vi "process-exe.vi"(0 "SR830 in":refnum<vi>, 1 "Monochromator":refnum<vi>, 3 "PowerGraph":refnum<vi>, 5 "Parameters":refnum<vi>, 9 "Process In":refnum<vi>, 11 "error in":errorcluster, 12 "Powermeter":refnum<vi>, 13 "Arr Power":refnum<vi>, 14 "Arr Refnum":refnum<vi>) -> (4 "Process out":refnum<vi>, 15 "error out":errorcluster)   [LabVIEW 2016]
uses:
  controls/process.ctl
  <vilib>/silver_ctls/ArrayMatrixCluster/Real Matrix NI_Silver.ctl
  <vilib>/Analysis/NI_AALBase.lvlib
panel:
  in  "PowerData":dbl[][](array[numeric])
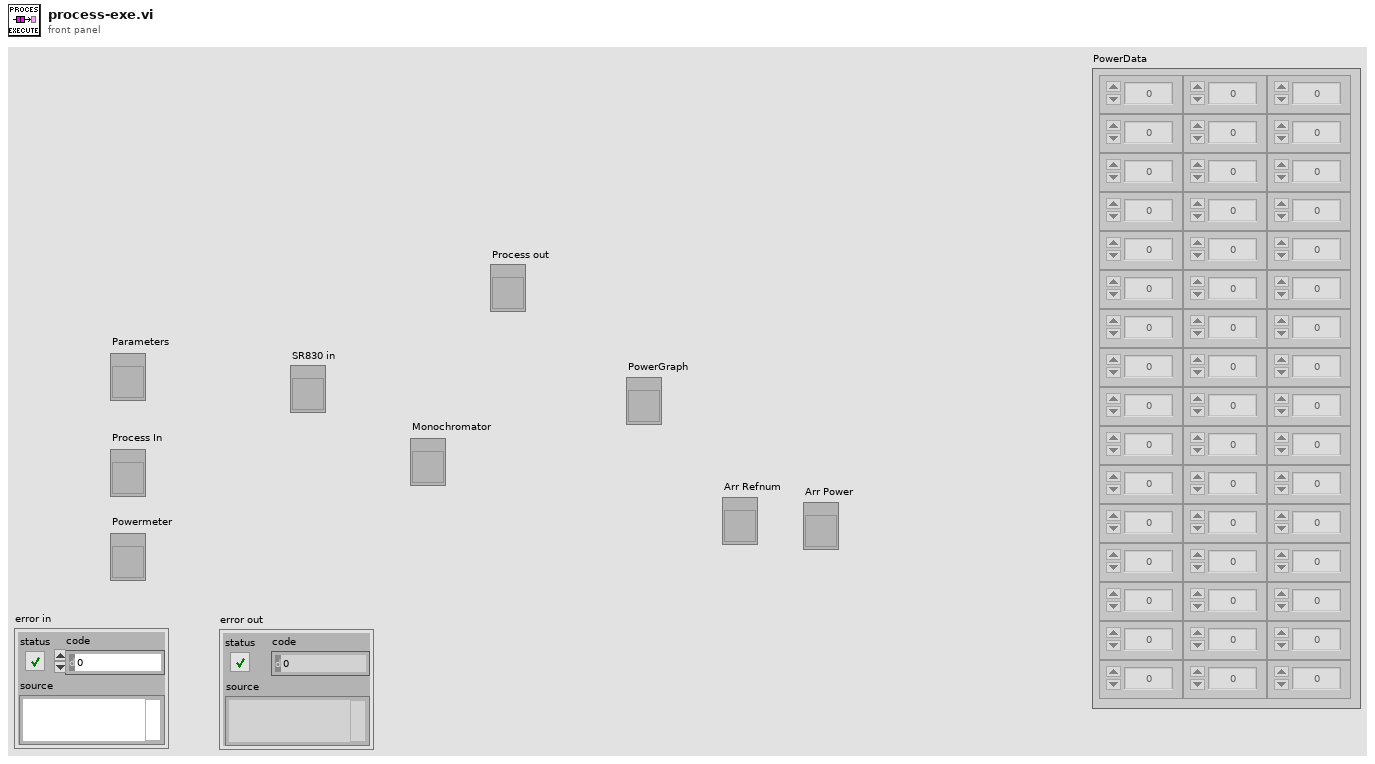
[diagram p1: front panel]
types:
  T1 = typedef "process.ctl" = cluster{"Sample":u16, "Lambda":u16, "Stabilizing":u16, "Status":u8, "Estimated Time":dbl, "Samples":T2, "Data":T2, "Lambda-Index":dbl, "Graph":bool}
  T2 = typedef "Real Matrix NI_Silver.ctl" = dbl[][]
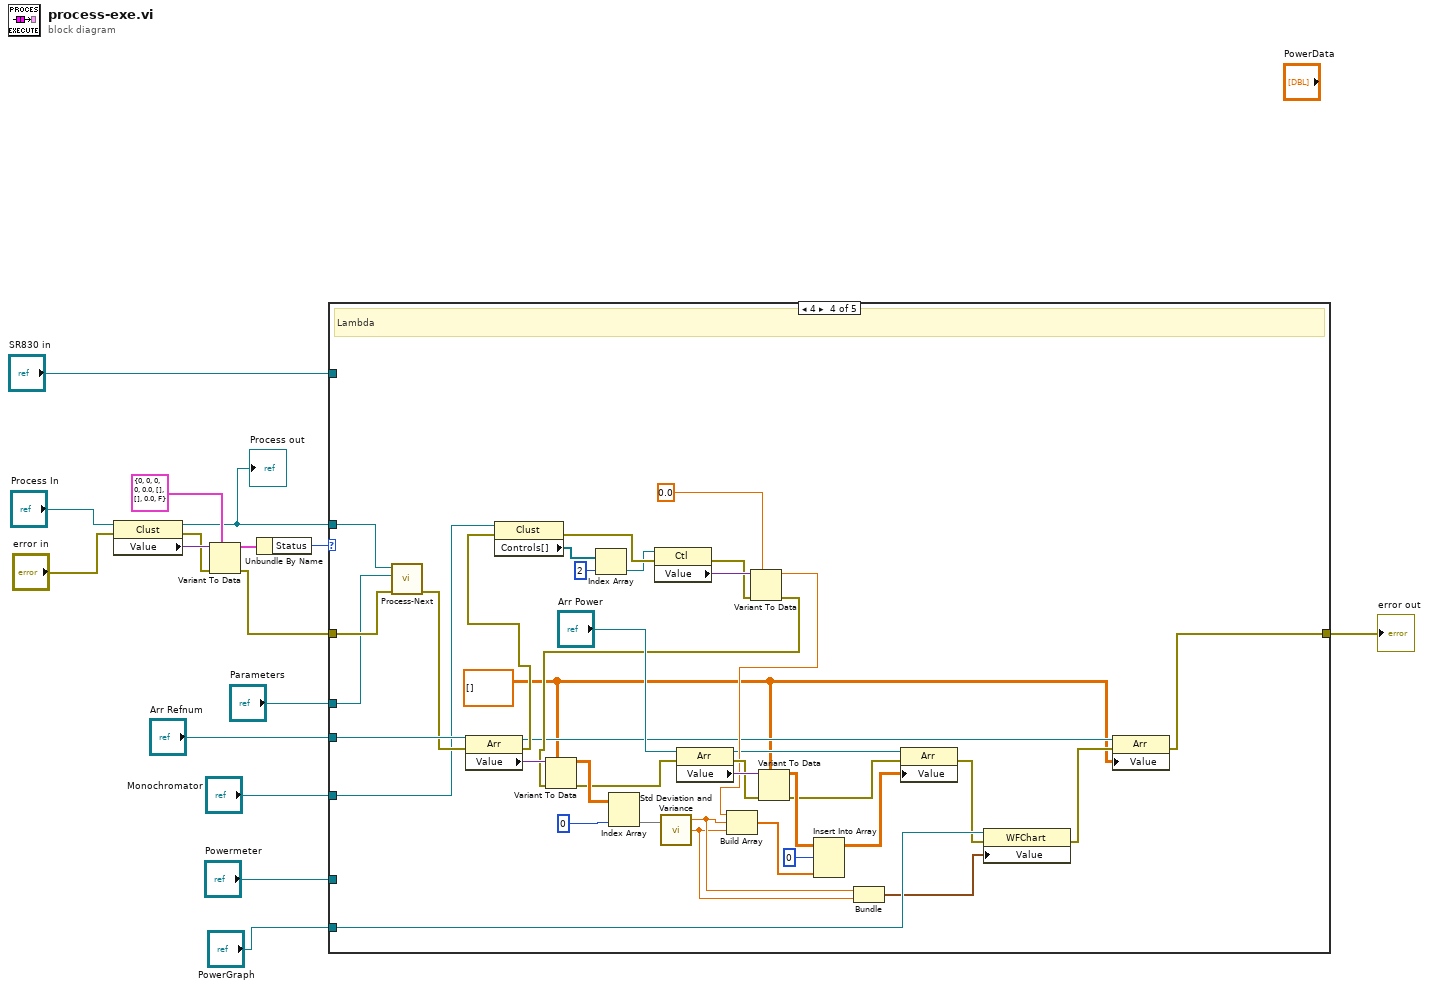
[diagram p0: block diagram]
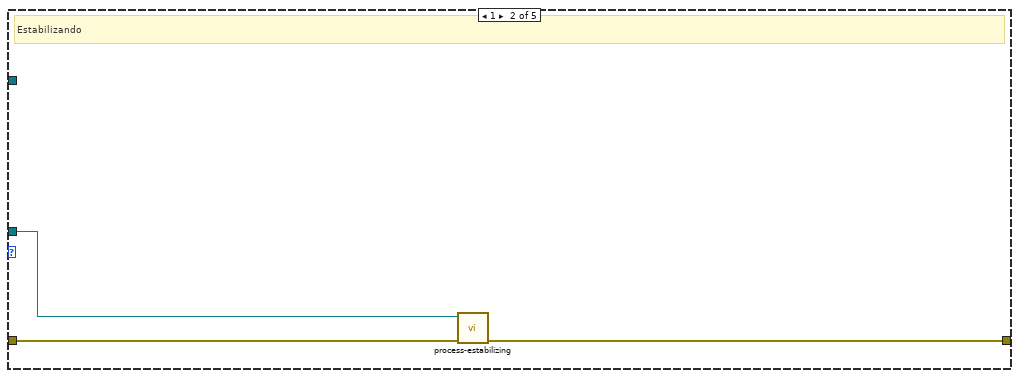
[diagram p3: hidden frame]
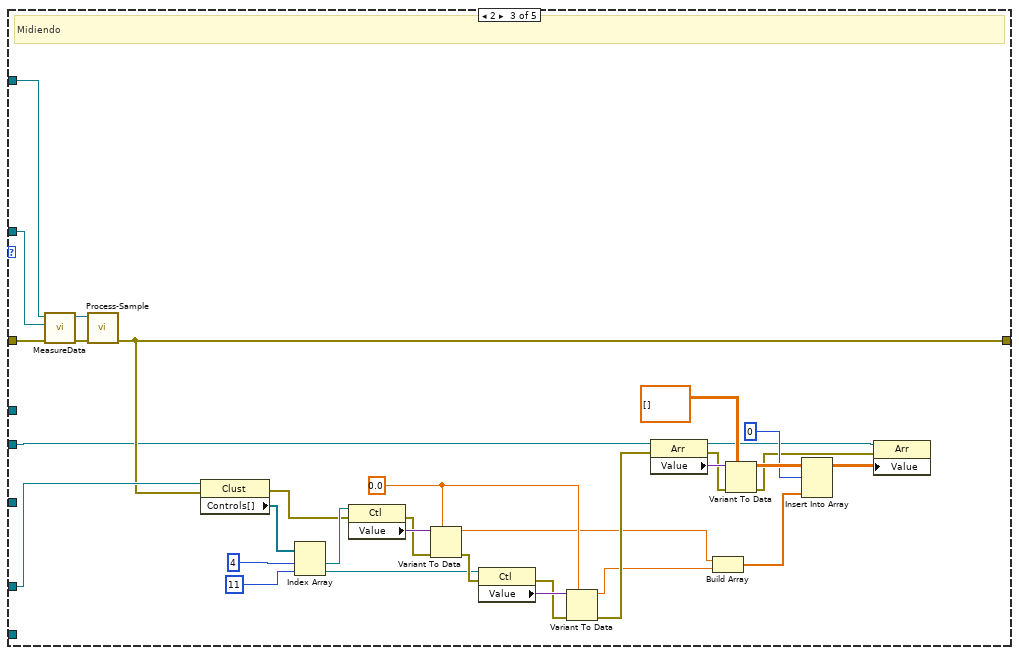
[diagram p4: hidden frame]
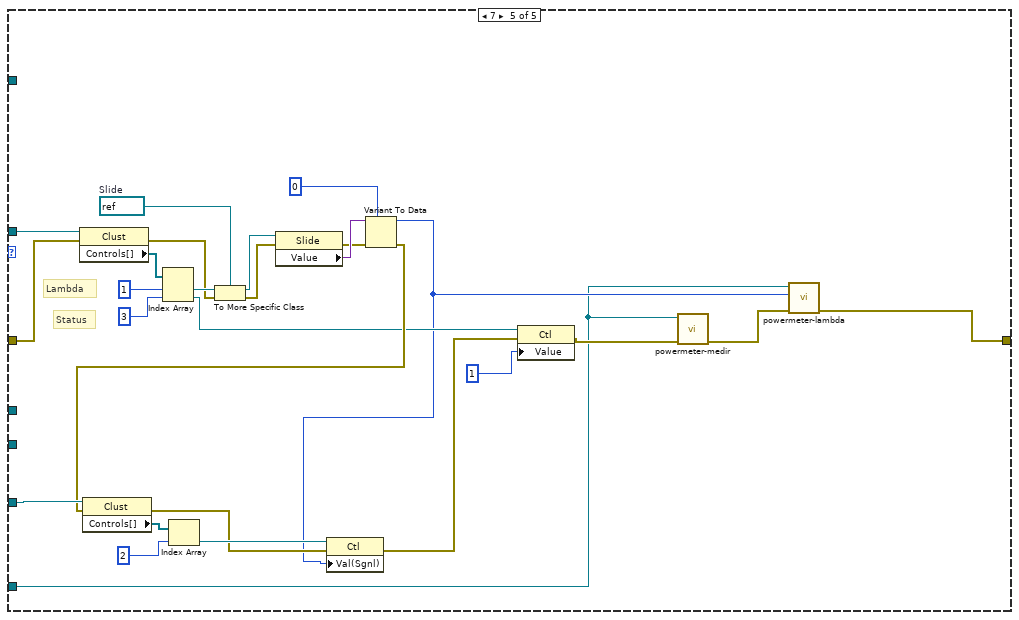
[diagram p5: hidden frame]
diagram:
  n1 = property class="Clust"(reference="Process In", error in="error in") -> (reference out=w7:refnum<vi>, error out=w13:errorcluster, "Value"=w14:variant)
  "Process out" <- w7
  n2 = Variant To Data(error in=w13, type=T1 {"Sample"=0, "Lambda"=0, "Stabilizing"=0, "Status"=0, "Estimated Time"=0.0, "Samples"=[], "Data"=[], "Lambda-Index"=0.0, "Graph"=FALSE} ("Process"), Variant=w14) -> (data=w11:T1, error out=w9:errorcluster)
  n3 = Unbundle By Name(w11) -> ("Status"=w10:u8)
  n4 = case shown="4" w10 {
    tunnel: w9 -> [w17 w20 w52 w91 w106]
    tunnel: [w17 w19 w46 w53 w96] -> w8
    tunnel: w7 -> [_ w18 w48 w65 w118]
    tunnel: "Parameters" -> [_ _ _ w90 _]
    tunnel: "SR830 in" -> [_ _ w49 _ _]
    tunnel: "Monochromator" -> [_ _ _ w66 w107]
    tunnel: "Powermeter" -> [_ _ w47 _ w92]
    tunnel: "Arr Refnum" -> [_ _ w33 w89 _]
    tunnel: "PowerGraph" -> [_ _ _ w61 _]
    frame 0, Default {
    }
    frame 1 {
      # "Estabilizando"
      n5 = call "process-estabilizing.vi"("error in (no error)"=w20, "Process in"=w18) -> ("error out"=w19:errorcluster)  [unwired: 9 in]
    }
    frame 2 {
      w35 = 0.0
      # "Midiendo"
      n6 = call "MeasureData.vi"("error in (no error)"=w52, "Process in"=w48, "SR830 in"=w49) -> ("Error Out"=w50:errorcluster, "Process out"=w51:refnum<vi>)  [unwired: 7 in]
      n7 = call "Process-Sample.vi"("error in (no error)"=w50, "Process"=w51) -> ("error out"=w46:errorcluster)  [unwired: 9 in]
      n8 = property class="Clust"(reference=w47, error in=w46) -> (error out=w41:errorcluster, "Controls[]"=w45:refnum<vi>[])  [unwired: 1 out]
      n9 = Index Array(array=w45, index #1=4 ("index"), index #2=11 ("index")) -> (element #1=w42:refnum<vi>, element #2=w37:refnum<vi>)
      n10 = property class="Ctl"(reference=w42, error in=w41) -> (error out=w39:errorcluster, "Value"=w40:variant)  [unwired: 1 out]
      n11 = Variant To Data(error in=w39, type=w35, Variant=w40) -> (data=w26:dbl, error out=w38:errorcluster)
      n12 = property class="Ctl"(reference=w37, error in=w38) -> (error out=w34:errorcluster, "Value"=w36:variant)  [unwired: 1 out]
      n13 = Variant To Data(error in=w34, type=w35, Variant=w36) -> (data=w25:dbl, error out=w32:errorcluster)
      n14 = property class="Arr"(reference=w33, error in=w32) -> (reference out=w23:refnum<vi>, error out=w29:errorcluster, "Value"=w31:variant)
      n15 = Build Array(w26, w25) -> (w24:dbl[])
      n16 = Variant To Data(error in=w29, type=dbl[][] [], Variant=w31) -> (data=w28:dbl[][], error out=w22:errorcluster)
      n17 = Insert Into Array(array=w28, index (row)=0 ("index"), new element=w24) -> (w21:dbl[][])  [unwired: 1 in]
      n18 = property class="Arr"(reference=w23, error in=w22, "Value"=w21) -> ()  [unwired: 2 out]
    }
    frame 4 {
      w54 = dbl[][] []
      # "Lambda"
      n19 = call "Process-Next.vi"("error in (no error)"=w91, "Parameters"=w90, "Process in"=w65) -> ("error out"=w88:errorcluster)  [unwired: 8 in]
      n20 = property class="Arr"(reference=w89, error in=w88) -> (reference out=w55:refnum<vi>, error out=w74:errorcluster, "Value"=w87:variant)
      n21 = property class="Clust"(reference=w66, error in=w74) -> (error out=w64:errorcluster, "Controls[]"=w76:refnum<vi>[])  [unwired: 1 out]
      n22 = Index Array(array=w76, index=2) -> (element=w63:refnum<vi>)
      n23 = property class="Ctl"(reference=w63, error in=w64) -> (error out=w71:errorcluster, "Value"=w73:variant)  [unwired: 1 out]
      n24 = Variant To Data(error in=w71, type=0.0, Variant=w73) -> (data=w69:dbl, error out=w70:errorcluster)
      n25 = Variant To Data(error in=w70, type=w54, Variant=w87) -> (data=w86:dbl[][], error out=w82:errorcluster)
      n26 = Index Array(array=w86, index (col)=0 ("disabled index (col)")) -> (element=w84:dbl[])  [unwired: 1 in]
      n27 = call <vilib>:"Std Deviation and Variance.vi"("X"=w84) -> ("mean"=w60:dbl, "standard deviation"=w59:dbl)  [unwired: 1 in, 1 out]
      n28 = property class="Arr"(reference="Arr Power", error in=w82) -> (reference out=w68:refnum<vi>, error out=w80:errorcluster, "Value"=w81:variant)
      n29 = Build Array(w69, w60, w59) -> (w77:dbl[])
      n30 = Variant To Data(error in=w80, type=w54, Variant=w81) -> (data=w79:dbl[][], error out=w62:errorcluster)
      n31 = Insert Into Array(array=w79, index (row)=0, new element=w77) -> (w67:dbl[][])  [unwired: 1 in]
      n32 = Bundle("mean"=w60, "standard deviation"=w59) -> (w58:cluster{"mean":dbl, "standard deviation":dbl})  [unwired: 1 in]
      n33 = property class="Arr"(reference=w68, error in=w62, "Value"=w67) -> (error out=w57:errorcluster)  [unwired: 1 out]
      n34 = property class="WFChart"(reference=w61, error in=w57, "Value"=w58) -> (error out=w56:errorcluster)  [unwired: 1 out]
      n35 = property class="Arr"(reference=w55, error in=w56, "Value"=w54) -> (error out=w53:errorcluster)  [unwired: 1 out]
    }
    frame 7 {
      w114 = refnum<vi> refnum  # Slide
      # "Status"
      # "Lambda"
      n36 = property class="Clust"(reference=w118, error in=w106) -> (error out=w113:errorcluster, "Controls[]"=w117:refnum<vi>[])  [unwired: 1 out]
      n37 = Index Array(array=w117, index #1=1 ("index"), index #2=3 ("index")) -> (element #1=w115:refnum<vi>, element #2=w99:refnum<vi>)
      n38 = To More Specific Class(target class=w114, reference=w115, error in=w113) -> (specific class reference=w112:refnum<vi>, error out=w111:errorcluster)
      n39 = property class="Slide"(reference=w112, error in=w111) -> (error out=w109:errorcluster, "Value"=w110:variant)  [unwired: 1 out]
      n40 = Variant To Data(error in=w109, type=0, Variant=w110) -> (data=w95:i32, error out=w105:errorcluster)
      n41 = property class="Clust"(reference=w107, error in=w105) -> (error out=w101:errorcluster, "Controls[]"=w104:refnum<vi>[])  [unwired: 1 out]
      n42 = Index Array(array=w104, index=2) -> (element=w102:refnum<vi>)
      n43 = property class="Ctl"(reference=w102, error in=w101, "Val(Sgnl)"=w95) -> (error out=w97:errorcluster)  [unwired: 1 out]
      n44 = property class="Ctl"(reference=w99, error in=w97, "Value"=1) -> (error out=w94:errorcluster)  [unwired: 1 out]
      n45 = call "powermeter-medir.vi"("error in (no error)"=w94, "Powermeter"=w92) -> ("error out"=w93:errorcluster)  [unwired: 9 in]
      n46 = call "powermeter-lambda.vi"("error in (no error)"=w93, "Lambda"=w95, "PowerMeter"=w92) -> ("error out"=w96:errorcluster)  [unwired: 7 in, 1 out]
    }
  }
  "error out" <- w8
